vi "IOTest.vi"() -> ()   [LabVIEW 2009]
panel:
  out "error out":errorcluster
  in  "stop":bool
  in  "DIO30":bool
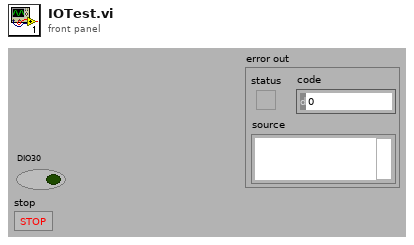
[diagram p1: front panel]
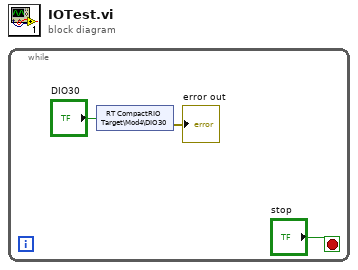
[diagram p0: block diagram]
diagram:
  n1 = while {
    stop <- "stop" stop-if-true
    n2 = shared-variable "RT CompactRIO Target\\Mod4\\DIO30"("DIO30") -> (error out=→"error out":errorcluster)  [unwired: 1 in]
  }
